vi "SEH Display Options to Saved Options.vi"(2 "Display Error Options":T3={"Code"="", "Shared Options"={"Number of Retries"=0, "Output Classification"="*Non-critical*", "Retry"=FALSE, "Classify Output"=FALSE, "Classify Notification"=FALSE, "Notification Classification"="*Non-critical*", "Convert Output to Warning"=FALSE, "Clear Output"=FALSE, "Notify"=FALSE, "Priority"=0, "Detect Warning"=FALSE, "Call VI"=FALSE, "VI to Call"="*Non-critical*"}}, 3 "Code":i32) -> (0 "Saved Error Options":T1={"Code"=0, "Shared Options"={"Number of Retries"=0, "Output Classification"="*Non-critical*", "Retry"=FALSE, "Classify Output"=FALSE, "Classify Notification"=FALSE, "Notification Classification"="*Non-critical*", "Convert Output to Warning"=FALSE, "Clear Output"=FALSE, "Notify"=FALSE, "Priority"=0, "Detect Warning"=FALSE, "Call VI"=FALSE, "VI to Call"="*Non-critical*"}})   [LabVIEW 2014]
uses:
  Controls/SEH/SEH Error Display Options.ctl
  Controls/SEH/SEH Shared Error Options.ctl
  Controls/SEH/SEH Error Options.ctl
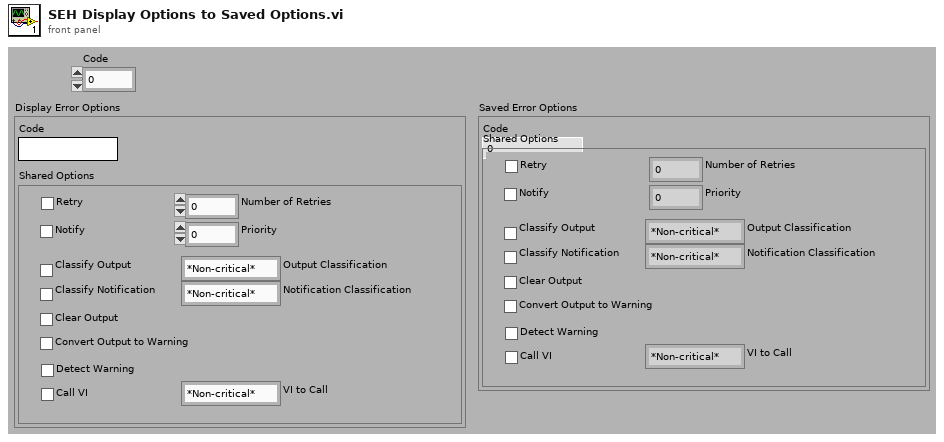
[diagram p1: front panel]
types:
  T1 = typedef "SEH Error Options.ctl" = cluster{"Code":i32, "Shared Options":T2}
  T2 = typedef "SEH Shared Error Options.ctl" = cluster{"Number of Retries":i32, "Output Classification":string, "Retry":bool, "Classify Output":bool, "Classify Notification":bool, "Notification Classification":string, "Convert Output to Warning":bool, "Clear Output":bool, "Notify":bool, "Priority":i32, "Detect Warning":bool, "Call VI":bool, "VI to Call":string}
  T3 = typedef "SEH Error Display Options.ctl" = cluster{"Code":string, "Shared Options":T2}
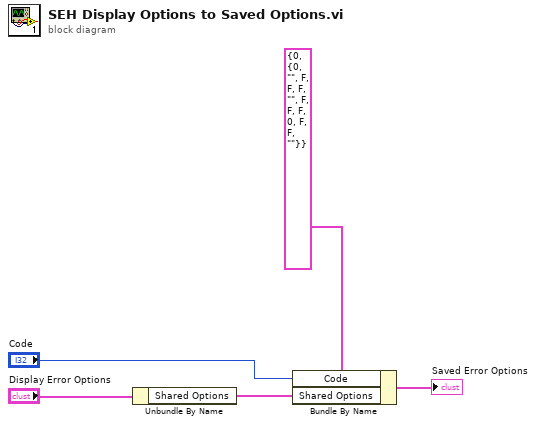
[diagram p0: block diagram]
diagram:
  n1 = Unbundle By Name("Display Error Options") -> ("Shared Options"=w2:T2)
  n2 = Bundle By Name(cluster=T1 {"Code"=0, "Shared Options"={"Number of Retries"=0, "Output Classification"="", "Retry"=FALSE, "Classify Output"=FALSE, "Classify Notification"=FALSE, "Notification Classification"="", "Convert Output to Warning"=FALSE, "Clear Output"=FALSE, "Notify"=FALSE, "Priority"=0, "Detect Warning"=FALSE, "Call VI"=FALSE, "VI to Call"=""}} ("Error Options 2"), "Code"="Code", "Shared Options"=w2) -> (→"Saved Error Options":T1)
